vi "Lechman_Target_A_1.vi"   [LabVIEW 2019]
uses:
  <vilib>/Platform/TimedLoop/XDataNode/timing_clust.ctl
  <vilib>/Platform/TimedLoop/XDataNode/nitl_modes.ctl
  <vilib>/Platform/TimedLoop/XDataNode/wakeup.ctl
  <vilib>/Platform/TimedLoop/XDataNode/XDataNode.xnode
  <vilib>/Platform/TimedLoop/XDataNode/XDNodeRunTimeDep.lvlib
types:
  T1 = typedef "XDNodeRunTimeDep.lvlib/timing_clust.ctl" = cluster{"Expected End [f-1]":u64, "Actual End [f-1]":u64, "Finished Late? [f-1]":bool, "Expected End [i-1]":u64, "Actual End [i-1]":u64, "Finished Late? [i-1]":bool, "Expected Start [i]":u64, "Actual Start [i]":u64, "Expected Start [f]":u64, "Actual Start [f]":u64, "Source Name":string, "Structure Name":string, "Period":i64, "Deadline":i64, "Offset":i64, "Start":i64, "Priority":i32, "Timeout":i32, "Mode":T2, "Wakeup Reason":T3, "Error":errorcluster, "Source Type":string, "Secondary Source Type":string, "Global End Time":u64, "Global Start Time":u64, "Frame Duration":u64, "Iteration Duration":u64, "Assigned CPU":i32, "I/O Scan Engine Mode":u32}
  T2 = typedef "XDNodeRunTimeDep.lvlib/nitl_modes.ctl" = enum32{"No Change", "Process missed periods, maintain original phase", "Discard missed periods, maintain original phase", "Process missed periods, ignore original phase", "Discard missed periods, ignore original phase"}
  T3 = typedef "XDNodeRunTimeDep.lvlib/wakeup.ctl" = enum32{"Normal", "Aborted", "Asynchronous wakeup", "Timing source error", "Timed loop error", "Timeout"}
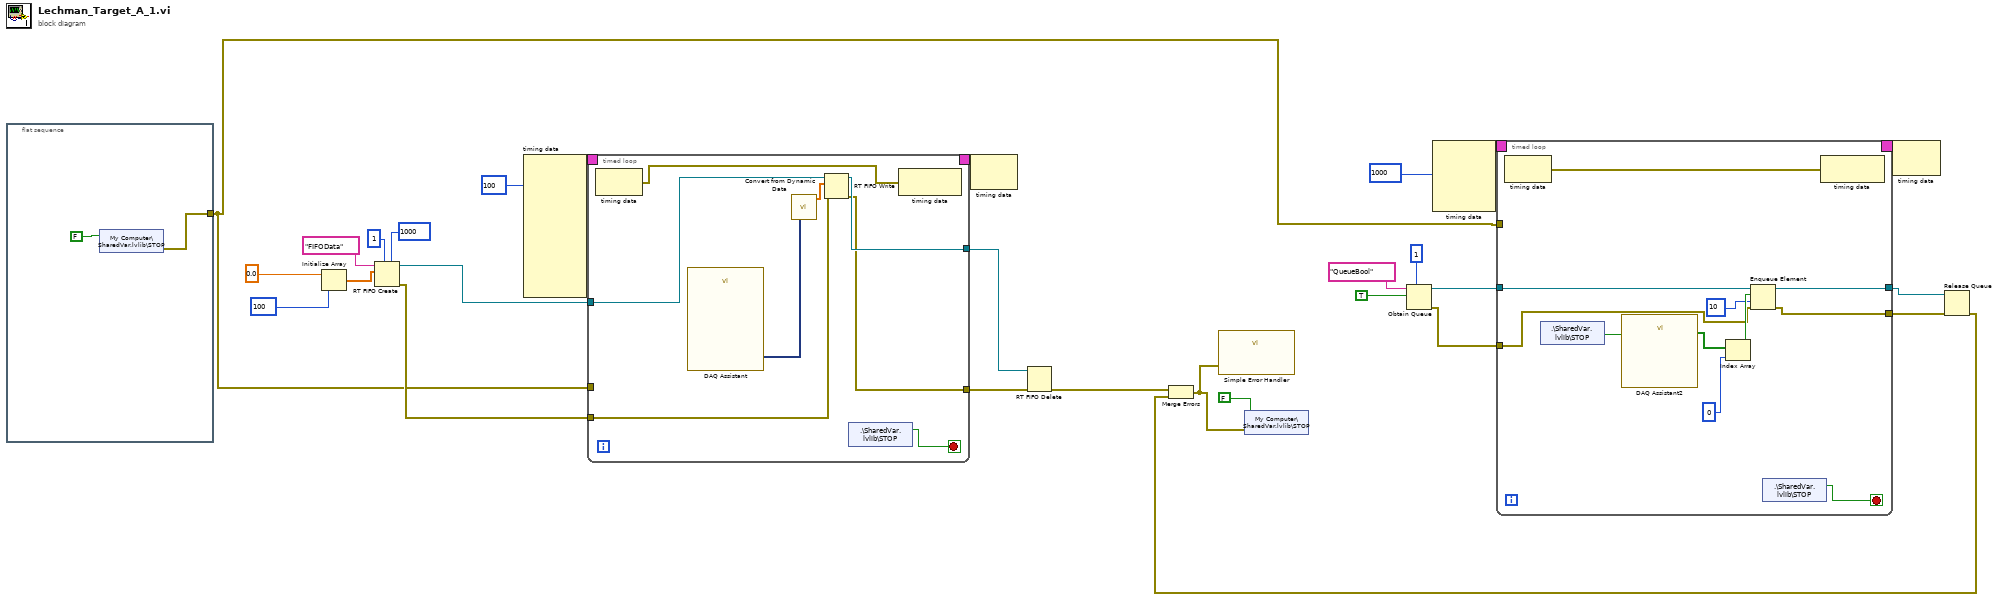
[diagram p0: block diagram]
diagram:
  n1 = flat-sequence {
    tunnel: [w29] -> w10
    frame #0 {
      n2 = shared-variable "My Computer\\SharedVar.lvlib\\STOP"(FALSE ("STOP")) -> (error out=w29:errorcluster)  [unwired: 1 in]
    }
  }
  n3 = Initialize Array(0.0, 100 ("dimension size")) -> (w23:dbl[])
  n4 = RT FIFO Create(0:"FIFOData" ("name (unnamed)"), 1:w23, 4:u32 1 ("size (10)"), 6:u32 1000 ("elements in array (1)")) -> (8:w28:refnum<k33>, 11:w27:errorcluster)  [unwired: 4 in, 1 out]
  n5 = node-c288(i64 100 ("Period")) -> (w20:T1)  [unwired: 9 in]
  n6 = timed-loop {
    timing: w20 -> [_]
    timing-out: [_] -> w19
    tunnel: w28 -> [w38]
    tunnel: [w36] -> w15
    tunnel: w27 -> [w33]
    tunnel: w10 -> [_]
    tunnel: [w32] -> w2
    stop <- w35 stop-if-true
    n7 = node-c288() -> (w31:errorcluster)  [unwired: 1 in]
    n8 = call "DAQ Assistant"() -> ("data"=w34:dynamicdata)  [unwired: 17 in, 2 out]
    n9 = call "Convert from Dynamic Data"("Dynamic Data Type"=w34) -> ("Array"=w37:dbl[])  [unwired: 3 in]
    n10 = RT FIFO Write(0:w38, 1:w37, 3:w33) -> (8:w36:refnum<k33>, 11:w32:errorcluster)  [unwired: 2 in, 2 out]
    n11 = shared-variable ".\\SharedVar.lvlib\\STOP"() -> (w35:bool)  [unwired: 1 in, 1 out]
    n12 = node-c288(w31) -> ()  [unwired: 1 out]
  }
  n13 = node-c288(w19) -> ()  [unwired: 1 out]
  n14 = RT FIFO Delete(0:w15, 3:w2) -> (11:w13:errorcluster)  [unwired: 1 in]
  n15 = Obtain Queue(max queue size (-1, unlimited)=1, name (unnamed)="QueueBool", element data type=TRUE) -> (queue out=w6:refnum<queue>, error out=w5:errorcluster)  [unwired: 2 in, 1 out]
  n16 = node-c288(i64 1000 ("Period")) -> (w18:T1)  [unwired: 3 in]
  n17 = timed-loop {
    timing: w18 -> [_]
    timing-out: [_] -> w17
    tunnel: w10 -> [_]
    tunnel: w6 -> [w54]
    tunnel: w5 -> [w46]
    tunnel: [w49] -> w4
    tunnel: [w45] -> w1
    stop <- w51 stop-if-true
    n18 = node-c288() -> (w44:errorcluster)  [unwired: 1 in]
    n19 = shared-variable ".\\SharedVar.lvlib\\STOP"() -> (w47:bool)  [unwired: 1 in, 1 out]
    n20 = call "DAQ Assistant2"("stop (T)"=w47) -> ("data"=w53:bool[])  [unwired: 16 in, 2 out]
    n21 = Index Array(array=w53, index=0) -> (element=w50:bool)
    n22 = Enqueue Element(queue=w54, element=w50, timeout in ms (-1)=10, error in (no error)=w46) -> (queue out=w49:refnum<queue>, error out=w45:errorcluster)  [unwired: 1 out]
    n23 = shared-variable ".\\SharedVar.lvlib\\STOP"() -> (w51:bool)  [unwired: 1 in, 1 out]
    n24 = node-c288(w44) -> ()  [unwired: 1 out]
  }
  n25 = node-c288(w17) -> ()  [unwired: 1 out]
  n26 = Release Queue(queue=w4, error in (no error)=w1) -> (error out=w3:errorcluster)  [unwired: 1 in, 2 out]
  n27 = Merge Errors(w13, w3) -> (w11:errorcluster)
  n28 = call <vilib>:"Simple Error Handler.vi"("error in (no error)"=w11) -> ()  [unwired: 4 in, 5 out]
  n29 = shared-variable "My Computer\\SharedVar.lvlib\\STOP"(FALSE ("STOP"), error in=w11) -> ()  [unwired: 1 out]
